vi "FTW-Actor-AddJob-NextConditional.vi"(2 "Add Next in Job Queue":string, 7 "FTW Actor Instance":refnum<class "FTW-ActorInstance.lvclass">, 13 "AddJob":bool=TRUE) -> (8 "FTW Actor Instance out":refnum<class "FTW-ActorInstance.lvclass">)   [LabVIEW 2015, in "FTW-ActorInstance.lvclass"]
uses:
  FTW-ActorInstance.lvclass
panel:
  # "Inputs"
  # "Outputs"
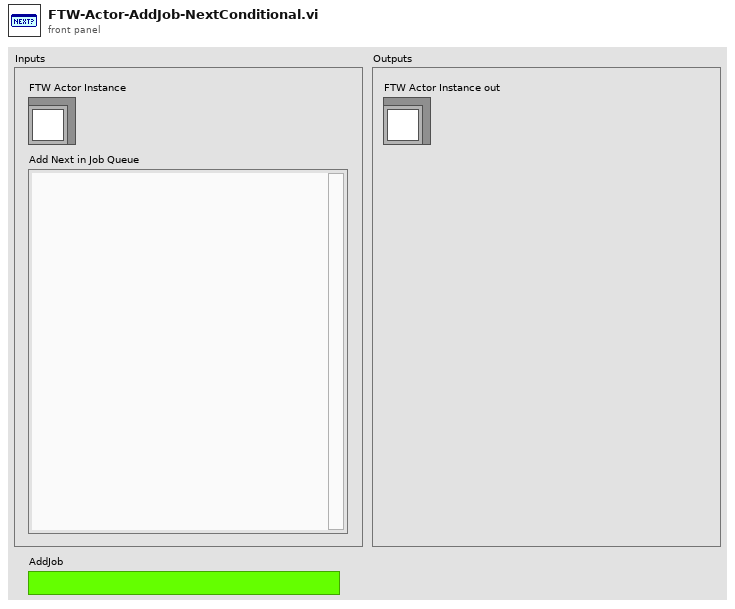
[diagram p1: front panel]
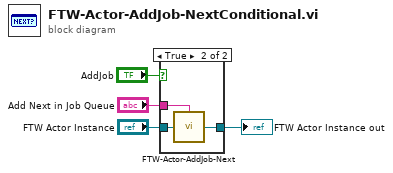
[diagram p0: block diagram]
diagram:
  n1 = case shown="True" "AddJob" {
    tunnel: "FTW Actor Instance" -> [w5 w8]
    tunnel: "Add Next in Job Queue" -> [_ w7]
    tunnel: [w5 w6] -> w2
    frame False {
    }
    frame True {
      n2 = call "FTW-Actor-AddJob-Next.vi"("Add Next in Job Queue"=w7, "FTW Actor Instance"=w8) -> ("FTW Actor Instance out"=w6:refnum<class "FTW-ActorInstance.lvclass">)  [unwired: 2 in]
    }
  }
  "FTW Actor Instance out" <- w2
